vi "stop.vi"(8 "error in (no error)":errorcluster, 11 "_cameraBase in":refnum<class "_cameraBase.lvclass">) -> (0 "error out":errorcluster, 3 "_cameraBase out":refnum<class "_cameraBase.lvclass">)   [LabVIEW 2019, in "_cameraBase.lvclass"]
uses:
  _cameraBase.lvclass
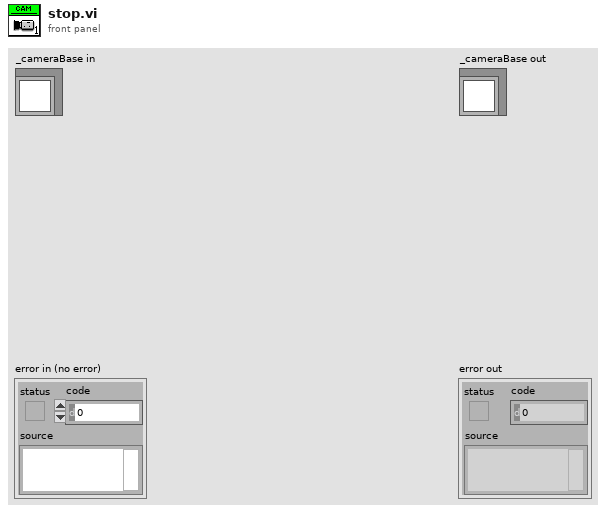
[diagram p1: front panel]
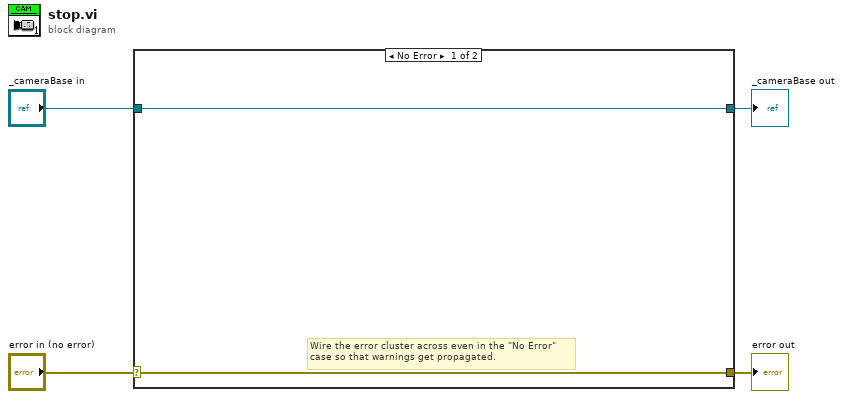
[diagram p0: block diagram]
diagram:
  n1 = case shown="No Error" "error in (no error)" {
    selector: "error in (no error)" -> [w5 w8]
    tunnel: [w5 w8] -> w3
    tunnel: [w6 w7] -> w1
    tunnel: "_cameraBase in" -> [w6 w7]
    frame No Error {
      # "Wire the error cluster across even in the \"No Error\"\ncase so that warnings get propagated."
    }
    frame Error {
    }
  }
  "error out" <- w3
  "_cameraBase out" <- w1
